vi "ColorReader.vi"(1 "file path (dialog if empty)":path=path "C:/Program Files (x86)/FRC Dashboard", 2 "name or relative path":string="Blue.csv") -> (0 "output cluster":T1)   [LabVIEW 2013]
uses:
  <vilib>/Utility/file.llb/Read From Spreadsheet File (string).vi
panel:
  out "LumMax":i32
  out "LumMin":i32
  out "SatMax":i32
  out "SatMin":i32
  out "HueMax":i32
  out "HueMin":i32
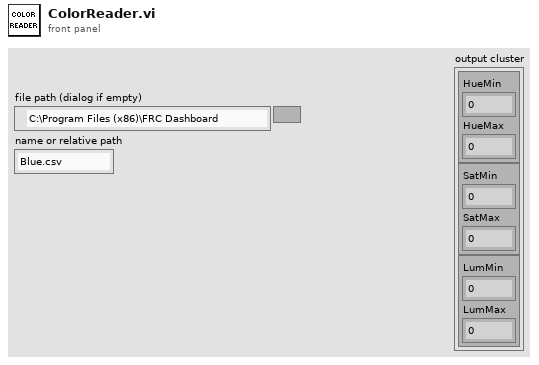
[diagram p1: front panel]
types:
  T1 = cluster{cluster{"HueMin":i32, "HueMax":i32}, cluster{"SatMin":i32, "SatMax":i32}, cluster{"LumMin":i32, "LumMax":i32}}
  T2 = cluster{"all rows[0]":string, "all rows[1]":string, "all rows[2]":string, "all rows[3]":string, "all rows[4]":string, "all rows[5]":string, "all rows[6]":string, "all rows[7]":string, "all rows[8]":string}
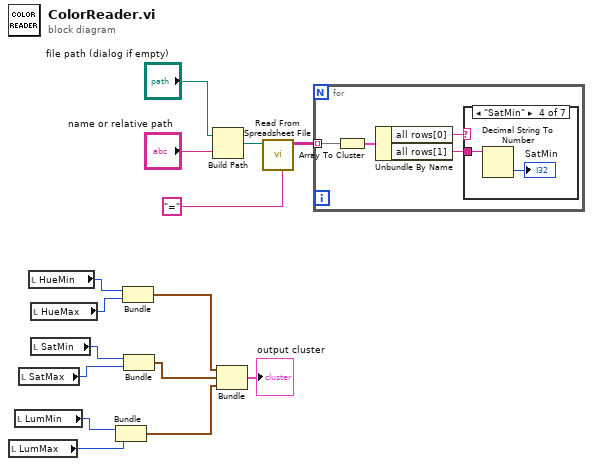
[diagram p0: block diagram]
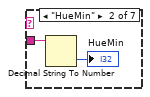
[diagram p3: hidden frame]
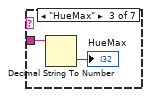
[diagram p4: hidden frame]
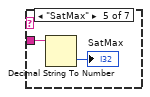
[diagram p5: hidden frame]
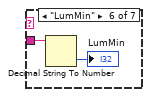
[diagram p6: hidden frame]
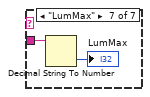
[diagram p7: hidden frame]
diagram:
  n1 = local read "LumMax"() -> (w5:i32)
  n2 = local read "LumMin"() -> (w6:i32)
  n3 = local read "SatMax"() -> (w7:i32)
  n4 = local read "HueMin"() -> (w10:i32)
  n5 = local read "HueMax"() -> (w9:i32)
  n6 = local read "SatMin"() -> (w8:i32)
  n7 = Bundle("LumMin"=w6, "LumMax"=w5) -> (w2:cluster{"LumMin":i32, "LumMax":i32})  [unwired: 1 in]
  n8 = Bundle("HueMin"=w10, "HueMax"=w9) -> (w4:cluster{"HueMin":i32, "HueMax":i32})  [unwired: 1 in]
  n9 = Bundle("SatMin"=w8, "SatMax"=w7) -> (w3:cluster{"SatMin":i32, "SatMax":i32})  [unwired: 1 in]
  n10 = Build Path(base path="file path (dialog if empty)", name or relative path="name or relative path") -> (appended path=w11:path)
  n11 = Bundle(w4, w3, w2) -> (→"output cluster":T1)  [unwired: 1 in]
  n12 = call-poly <vilib>:"Read From Spreadsheet File.vi"("delimiter (\\t)"="=", "file path (dialog if empty)"=w11) -> ("all rows"=w12:string[][])  [unwired: 5 in, 4 out]
  n13 = for {
    tunnel: w12 -> [w19] mode=indexing
    n14 = Array To Cluster(array=w19) -> (cluster=w18:T2)
    n15 = Unbundle By Name(w18) -> ("all rows[0]"=w17:string, "all rows[1]"=w16:string)
    n16 = case shown="\"SatMin\"" w17 {
      tunnel: w16 -> [_ w21 w23 w25 w27 w29 w31]
      frame "", Default {
      }
      frame "HueMin" {
        n17 = Decimal String To Number(string=w21) -> (number=→"HueMin":i32)  [unwired: 2 in, 1 out]
      }
      frame "HueMax" {
        n18 = Decimal String To Number(string=w23) -> (number=→"HueMax":i32)  [unwired: 2 in, 1 out]
      }
      frame "SatMin" {
        n19 = Decimal String To Number(string=w25) -> (number=→"SatMin":i32)  [unwired: 2 in, 1 out]
      }
      frame "SatMax" {
        n20 = Decimal String To Number(string=w27) -> (number=→"SatMax":i32)  [unwired: 2 in, 1 out]
      }
      frame "LumMin" {
        n21 = Decimal String To Number(string=w29) -> (number=→"LumMin":i32)  [unwired: 2 in, 1 out]
      }
      frame "LumMax" {
        n22 = Decimal String To Number(string=w31) -> (number=→"LumMax":i32)  [unwired: 2 in, 1 out]
      }
    }
  }
